vi "读取寄存器(子VI).vi"(6 "error in (no error)":errorcluster caption="错误输入（无错误）", 7 "baud rate (9600)":u32=9600 caption="波特率(9600)", 8 "number of holding registers":u16 caption="保持寄存器数量", 9 "starting address":u16 caption="起始地址", 10 "unit ID":u8=1 caption="单元ID", 11 "VISAResourceName输入":refnum<vi>) -> (3 "register values":u16[](array[numeric]) caption="寄存器值", 4 "error out":errorcluster caption="错误输出")   [LabVIEW 2016, in "斯坦道CODMn.lvlib"]
uses:
  <vilib>/Modbus/master/Create Master Instance (Serial).vi
  <vilib>/Modbus/master/Modbus Master.lvclass
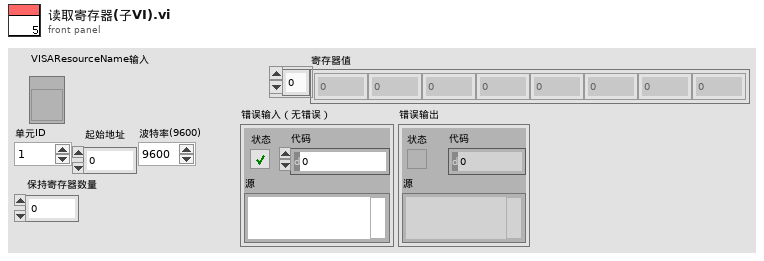
[diagram p1: front panel]
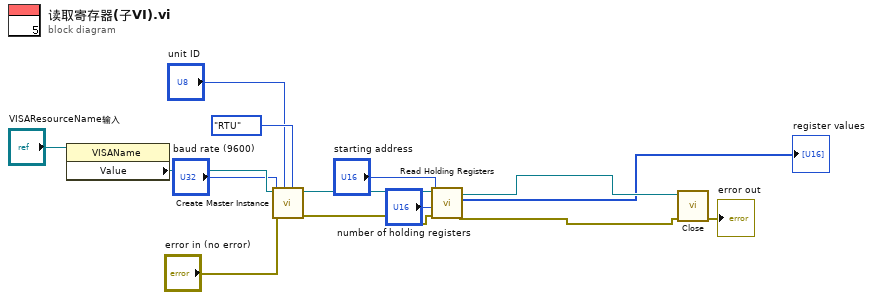
[diagram p0: block diagram]
diagram:
  n1 = property class="VISAName"(reference="VISAResourceName输入") -> ("Value"=w13:refnum<visa-resource-name>)  [unwired: 1 in, 2 out]
  n2 = call-poly <vilib>:"Create Master Instance.vi"("serial type"=enum16{"RTU", "ASCII"}."RTU", "unit ID"="unit ID", "error in (no error)"="error in (no error)", "baud rate (9600)"="baud rate (9600)", "VISA resource name"=w13) -> ("error out"=w9:errorcluster, "serial master instance"=w8:refnum<class "Modbus Master.lvclass">)  [unwired: 5 in]
  n3 = call-dynamic "Read Holding Registers.vi"("error in (no error)"=w9, "number of holding registers"="number of holding registers", "starting address"="starting address", "Modbus master in"=w8) -> ("error out"=w12:errorcluster, "register values"=→"register values":u16[], "Modbus master out"=w11:refnum<class "Modbus Master.lvclass">)  [unwired: 5 in]
  n4 = call-dynamic "Close.vi"("error in (no error)"=w12, "Modbus master in"=w11) -> ("error out"=→"error out":errorcluster)  [unwired: 9 in]
